vi "get boat location.vi"(9 "Tug":string="L", 11 "Nav String":string="$,G,43,13,230,P,10,20,120,T,10,10,330,L,14,36,110,A,3,5,B,7,8,C,16,20,D,-1,-1,S,08,12,234\r") -> (0 "Valid ?":bool, 1 "angle":i32, 2 "y":i32, 3 "x":i32)   [LabVIEW 2013]
doc: "This VI gets the location for the Tug specified along with the time data for the data. The output cluster has which boat it is, x, y, and angle, in that order."
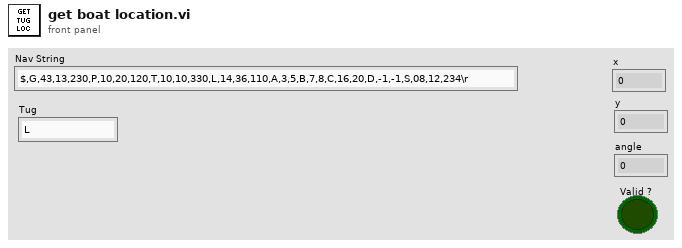
[diagram p1: front panel]
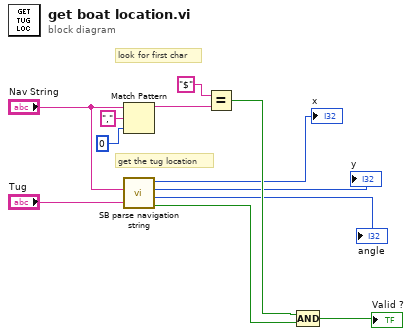
[diagram p0: block diagram]
diagram:
  # "get the tug location"
  # "look for first char"
  n1 = Match Pattern(string="Nav String", regular expression=",", offset (0)=0) -> (before substring=w11:string)  [unwired: 3 out]
  n2 = call "SB parse navigation string.vi"("Header"="Tug", "Nav String"="Nav String") -> ("Valid?"=w6:bool, "angle"=→"angle":i32, "y"=→"y":i32, "x"=→"x":i32)  [unwired: 4 in]
  n3 = Equal?(x="$", y=w11) -> (x = y?=w7:bool)
  n4 = Compound Arithmetic op=AND(w7, w6) -> (→"Valid ?":bool)
